vi "MPU6050 Private class data.vi"() -> ()   [LabVIEW 2017]
panel:
  in  "Bias":cluster{"X":dbl, "Y":dbl, "Z":dbl}
  in  "Address":u8=104 format="%x"
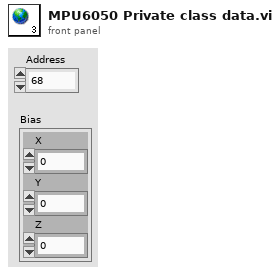
[diagram p1: front panel]
diagram:
